vi "FGV FT-IR Kalibrieren.vi"(10 "Aktionen FT-IR Kalibrieren":T1, 11 "Sprachliste":string[][](array[string])) -> (1 "Zustand FT-IR":string, 2 "Aktionen FT-IR Kalibrieren":T1)   [LabVIEW 2020, in "Auto Kalibrieren.lvlib"]
uses:
  Auto Kalibrieren.lvlib
  Aktionen FT-IR Kalibrieren.ctl
  Seiten/FT-IR/FGV FT-IR Aktionen.ctl
  Seiten/FT-IR/FGV FT-IR Gasliste Aktionen.ctl
  Aktion FGV CalZustand.ctl
  Stoerungen/Stoerungen Messgeraet/Aktionen Kommunikation Stoerung.ctl
  Aktionen FGV Zustand Kalibrierung.ctl
  Messdaten/Aktionen FGV Messdaten.ctl
  Schedule Modul/Aktion FGV Testdaten sammeln.ctl
  Seiten/FT-IR/TOOLweb Interface Library/Trigger Aktionen.ctl
  Seiten/FT-IR/ReadLabFile/Aktionen Lab File.ctl
  Seiten/FT-IR/FT-IR.lvlib
  Allgemein/allgemeine Sub-VIs.lvlib
  Stoerungen/Stoerungen.lvlib
  Seiten/FT-IR/TOOLweb Interface Library/Typdefinitionen.lvlib
  Seiten/FT-IR/TOOLweb Interface Library/TOOLweb Interface.lvlib
  Messdaten/Messdaten.lvlib
  Seiten/FT-IR/ReadLabFile/Read Lab File.lvlib
  Sprachverwaltung/Sprachverwaltung.lvlib
  Schedule Modul/Schedule Modul.lvlib
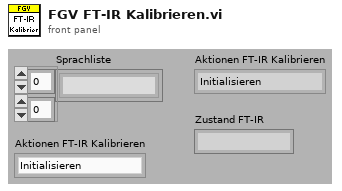
[diagram p1: front panel]
types:
  T1 = typedef "Auto Kalibrieren.lvlib/Aktionen FT-IR Kalibrieren.ctl" = enum16{"Initialisieren", "Anstehende Störung", "CO2, H2O - Vergleichen", "Hintergrund starten", "Hintergrund", "Hintergrund Abgeschlossen", "Fertig", "Beenden"}
  T2 = typedef "Auto Kalibrieren.lvlib/Aktion FGV CalZustand.ctl" = enum16{"lesen", "Cal FTIR", "Cal FID CH4", "Cal PMA", "init", "Cal FID THC", "THC CG Eingang"}
  T3 = typedef "FT-IR.lvlib/FGV FT-IR Gasliste Aktionen.ctl" = enum16{"lesen", "Gasliste FT-IR", "Gasliste ausgelesen", "laden", "speichern", "löschen"}
  T4 = typedef "FT-IR.lvlib/FGV FT-IR Aktionen.ctl" = enum16{"lesen", "NOG setzen", "NOS setzen", "Initialisieren", "speichern", "ALLES setzen", "FT-IR Spektrum loggen", "Komm Stoppen", "Spektrum LogKonfig"}
  T5 = typedef "Stoerungen.lvlib/Aktionen Kommunikation Stoerung.ctl" = enum16{"lesen", "init", "FT-IR Komm", "FT-IR Betriebsart", "FT-IR Hintergrund", "cRIO Komm", "PNS Komm", "Dichtheitstest", "Life Bit", "FTIR Komm AK", "PMA Komm", "FID Komm", "PMA Cal", "FID Ch4 Cal", "FID THC Cal", "Cal Timeout", "VFS 1 Komm", "VFS 2 Komm", "VFS 3 Komm", "VFS 4 Komm", "TRE 08 Komm", "CG-Test vorzeitig", "CG-Test Span 1", "CG-Test Span 2", "CG-Test Span 3", "CG-Test Messgas", "CG-Test löschen", "Test", "Amium AK", "AK Recept konfig", "AK Name konfig", "AK EKFG konfig"}
  T6 = typedef "Auto Kalibrieren.lvlib/Aktionen FGV Zustand Kalibrierung.ctl" = enum16{"lesen", "LÖSCHEN", "Hintergrund fertig", "Nullpunkt NDIR CO lo", "Endpunkt NDIR CO lo", "Nullpunkt NDIR CO hi", "Endpunkt NDIR CO hi", "Nullpunkt NDIR CO2 lo", "Endpunkt NDIR CO2 lo", "Nullpunkt FID CH4", "Endpunkt FID CH4", "Nullpunkt FID THC", "Endpunkt FID THC", "Nullpunkt PMA", "Endpunkt PMA", "Fehler FT-IR", "Fehler NDIR lo", "Fehler FID CH4", "Fehler FID THC", "Fehler PMA", "TIMEOUT"}
  T7 = typedef "Messdaten.lvlib/Aktionen FGV Messdaten.ctl" = enum16{"lesen", "schreiben", "löschen", "Mittelwerte", "Komponente"}
  T8 = typedef "Schedule Modul.lvlib/Aktion FGV Testdaten sammeln.ctl" = enum16{"lesen", "Dichtheitstest", "CalGasTest", "T90", "Kalibrieren", "init", "Kalender Daten"}
  T9 = typedef "FT-IR.lvlib/TOOLweb Interface.lvlib/Typdefinitionen.lvlib/Trigger Aktionen.ctl" = enum16{"startrun", "runonce", "stoprun", "pauserun", "resumerun", "takeback"}
  T10 = typedef "FT-IR.lvlib/Read Lab File.lvlib/Aktionen Lab File.ctl" = enum16{"lesen", "laden"}
  T11 = typedef "String - Ausgabefeld.ctl" = string
  T12 = typedef "Stoerungen.lvlib/Stoerungen Messgeraete.ctl" = cluster{"FT-IR Komm":bool, "FT-IR Betriebsart":bool, "FT-IR Hintergrundscan":bool, "Dichtheitstest":bool, "cRIO Komm":bool, "PNS Komm":bool, "Life Bit":bool, "FT-IR AK Komm":bool, "PMA Komm":bool, "FID Komm":bool, "PMA Cal":bool, "FID CH4 Cal":bool, "FID THC Cal":bool, "Cal Timeout":bool, "VFS 1 Komm":bool, "VFS 2 Komm":bool, "VFS 3 Komm":bool, "VFS 4 Komm":bool, "TRE 08 Komm":bool, "CG-Test":bool, "CG-Test 1":bool, "CG-Test 2":bool, "CG-Test 3":bool, "Messgas - Eingang":bool, "Amium AK Komm":bool, "AK Rezept nicht konfiguriert ":bool, "AK Name nicht konfiguriert":bool, "AK EKFG nicht konfiguriert":bool}
  T13 = typedef "Schedule Modul.lvlib/Ergebnis Kalibrieren.ctl" = cluster{"Fehler":bool, "CO2 H2O vergleich":bool}
  T14 = typedef "Auto Kalibrieren.lvlib/Zustand Messgeraete Kalibrierung.ctl" = cluster{"Hintergrund FT-IR":bool, "Nullpunkt NDIR CO lo":bool, "Endpunkt NDIR CO lo":bool, "Nullpunkt NDIR CO hi":bool, "Endpunkt NDIR CO hi":bool, "Nullpunkt NDIR CO2 lo":bool, "Endpunkt NDIR CO2 lo":bool, "Nullpunkt FID CH4":bool, "Endpunkt FID CH4":bool, "Nullpunkt FID THC":bool, "Endpunkt FID THC":bool, "Nullpunkt PMA":bool, "Endpunkt PMA":bool, "Fehler FT-IR":bool, "Fehler NDIR lo":bool, "Fehler FID CH4":bool, "Fehler FID THC":bool, "Fehler PMA":bool}
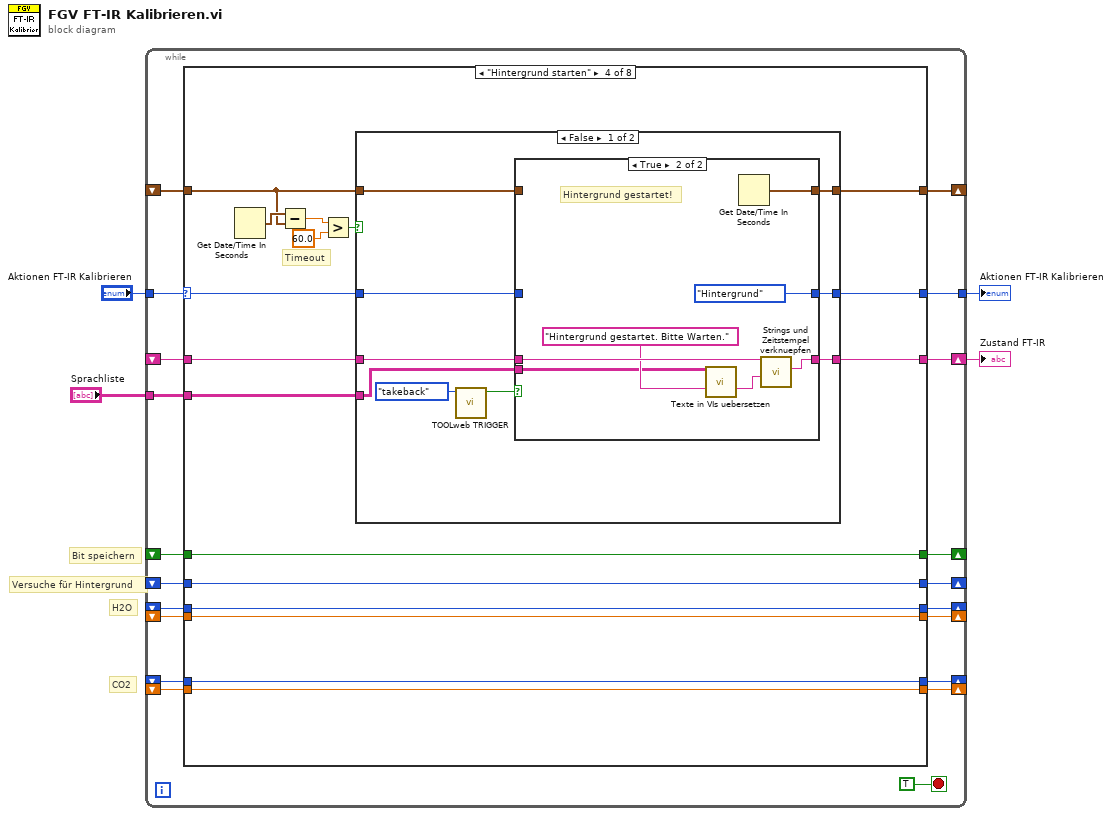
[diagram p0: block diagram]
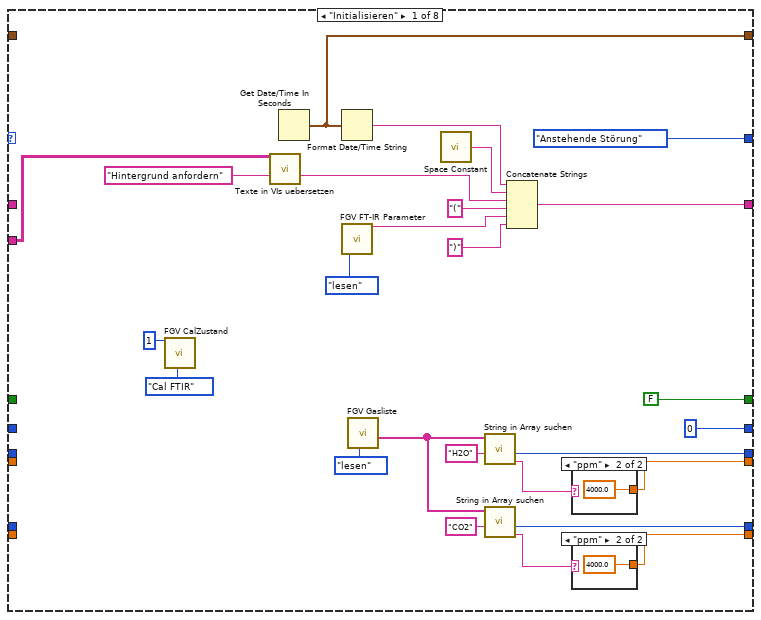
[diagram p2: hidden frame]
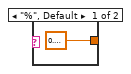
[diagram p3: hidden frame]
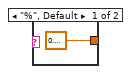
[diagram p4: hidden frame]
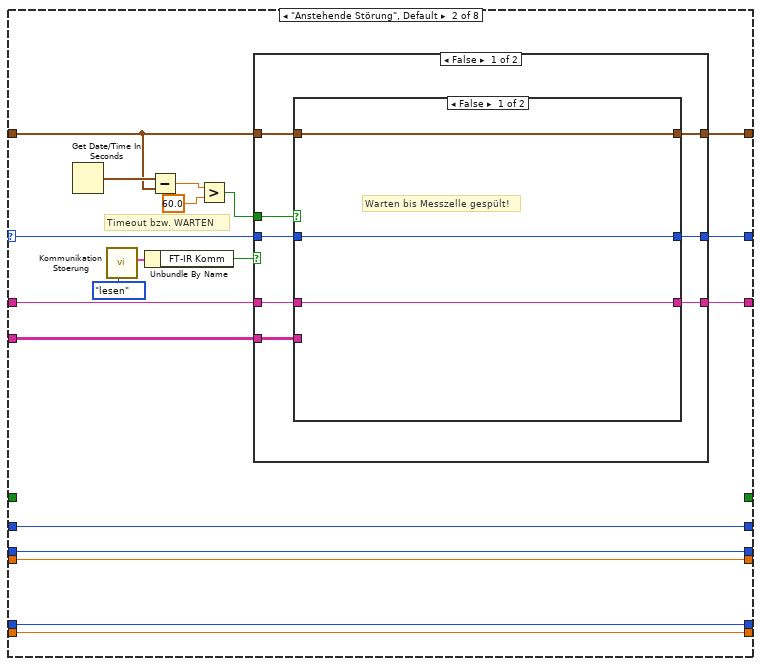
[diagram p5: hidden frame]
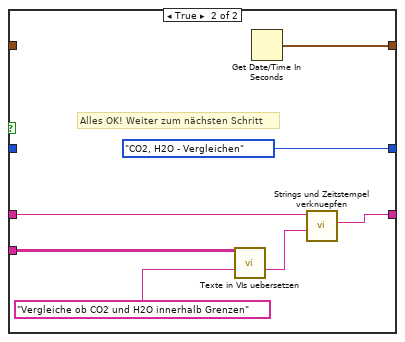
[diagram p6: hidden frame]
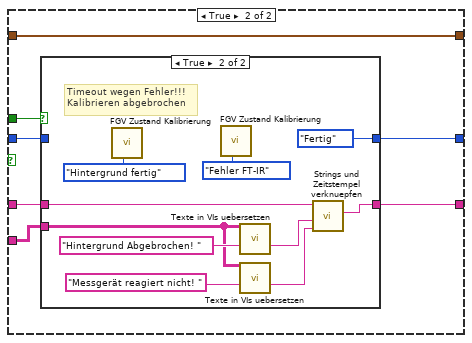
[diagram p7: hidden frame]
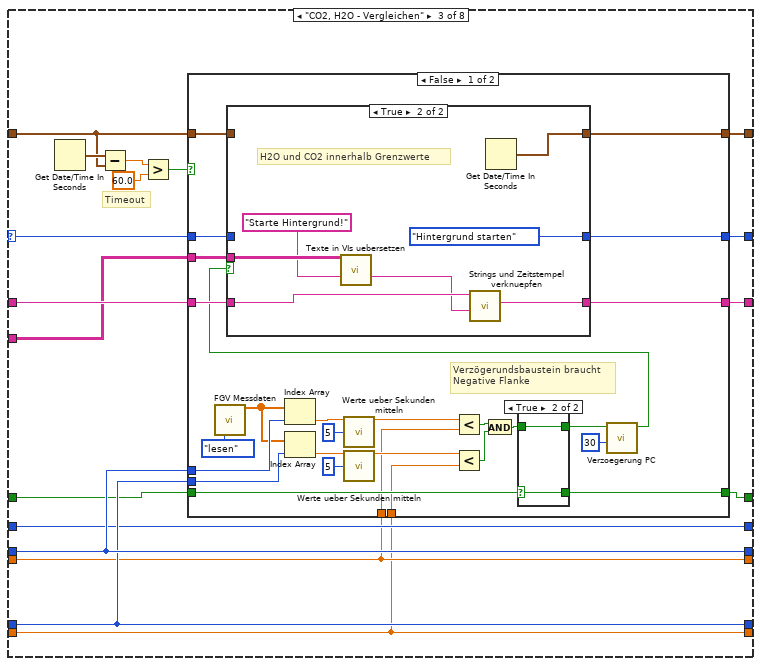
[diagram p9: hidden frame]
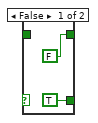
[diagram p10: hidden frame]
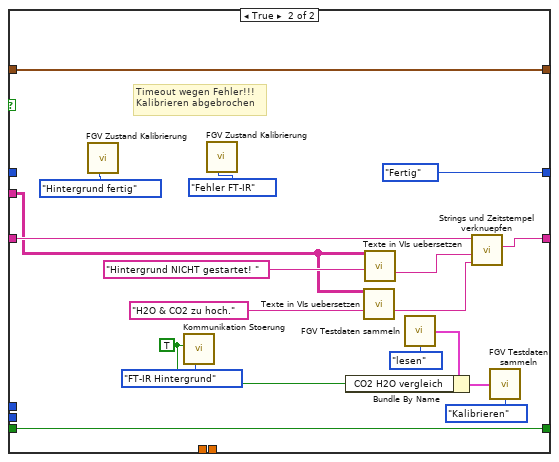
[diagram p12: hidden frame]
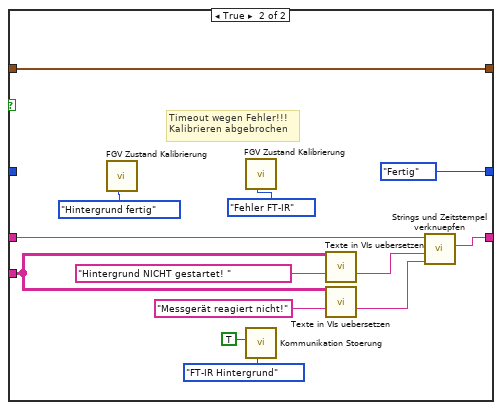
[diagram p14: hidden frame]
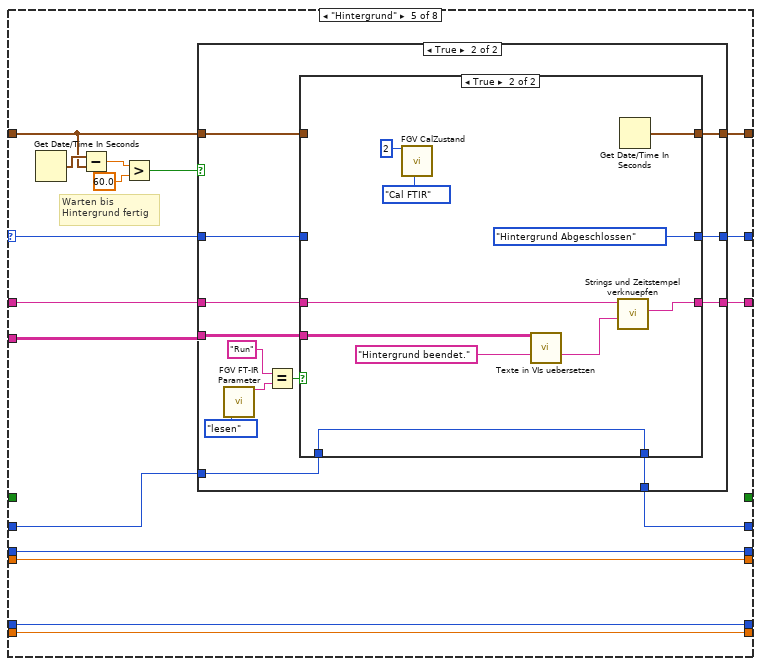
[diagram p15: hidden frame]
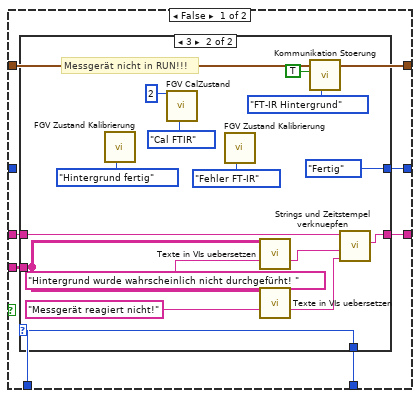
[diagram p17: hidden frame]
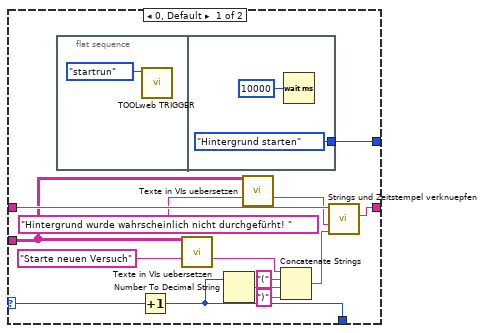
[diagram p18: hidden frame]
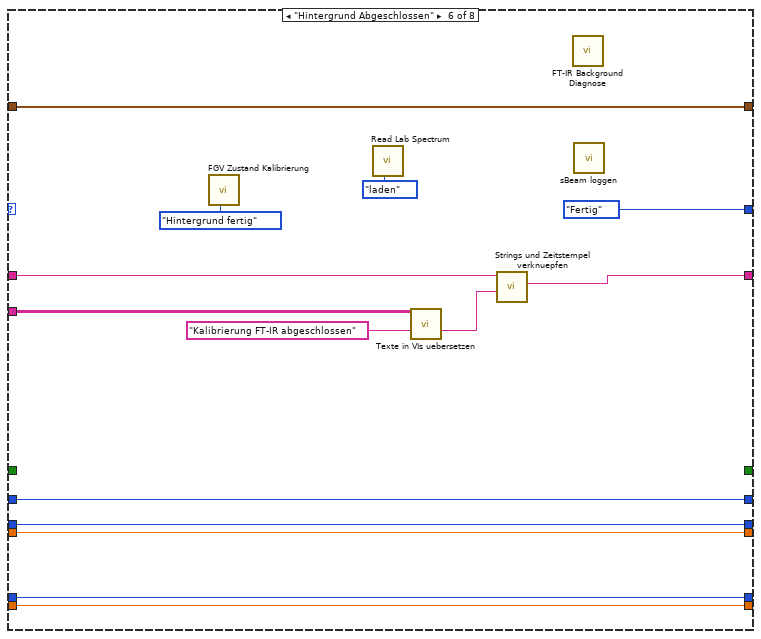
[diagram p19: hidden frame]
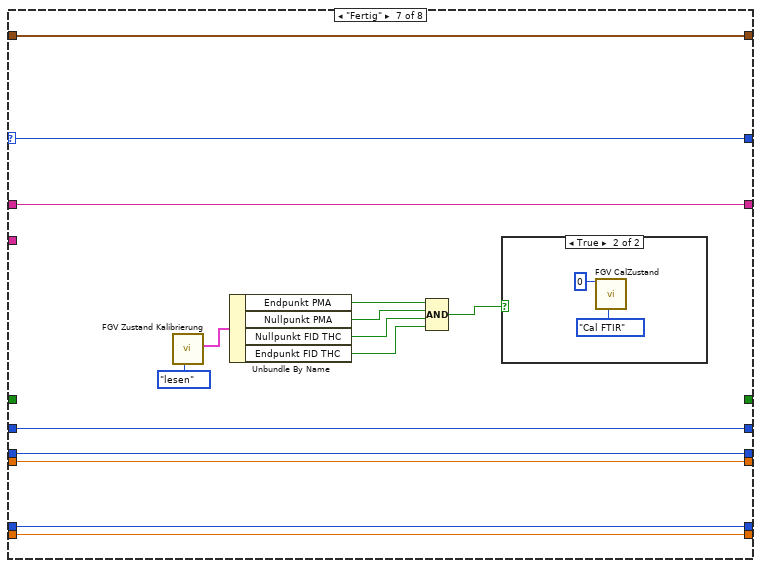
[diagram p20: hidden frame]
diagram:
  # "CO2"
  # "H2O"
  # "Versuche für Hintergrund"
  # "Bit speichern"
  n1 = while {
    shift-right: [w22] -> _
    shift-left: _ -> [w23]
    shift-right: [w18] -> w4
    shift-left: _ -> [w17]
    shift-right: [w15] -> _
    shift-left: _ -> [w20]
    shift-right: [w16] -> _
    shift-left: _ -> [w19]
    tunnel: "Aktionen FT-IR Kalibrieren" -> [w24]
    tunnel: [w21] -> w3
    shift-right: [w12] -> _
    shift-left: _ -> [w13]
    shift-right: [w11] -> _
    shift-left: _ -> [w10]
    tunnel: "Sprachliste" -> [w9]
    shift-right: [w8] -> _
    shift-left: _ -> [w7]
    shift-right: [w6] -> _
    shift-left: _ -> [w5]
    stop <- TRUE stop-if-true
    n2 = case shown="\"Hintergrund starten\"" w24 {
      selector: w24 -> [_ w66 w119 w195 w244 _ w347 _]
      tunnel: w23 -> [_ w62 w121 w196 w247 w332 w348 _]
      tunnel: [w43 w61 w120 w197 w246 w332 w348 w354] -> w22
      tunnel: [Aktionen_FT-IR_Kalibrieren."Anstehende Störung" ("Aktionen FT-IR Kalibrieren") w67 w124 w200 w248 Aktionen_FT-IR_Kalibrieren."Fertig" ("Aktionen FT-IR Kalibrieren") w347 Aktionen_FT-IR_Kalibrieren."Fertig" ("Aktionen FT-IR Kalibrieren")] -> w21
      tunnel: w17 -> [_ w64 w123 w199 w249 w331 w346 _]
      tunnel: [w42 w63 w122 w198 w245 w330 w346 "" ("Verknüpfter String")] -> w18
      tunnel: w20 -> [_ w60 w118 w194 w241 w329 w345 w358]
      tunnel: w19 -> [_ w59 w117 w193 w240 w328 w344 w357]
      tunnel: [w29 w59 w117 w193 w240 w328 w344 w357] -> w16
      tunnel: [w30 w60 w118 w194 w241 w329 w345 w358] -> w15
      tunnel: w13 -> [_ _ w116 w192 _ _ _ _]
      tunnel: [FALSE _ w115 w192 _ _ _ _] -> w12
      tunnel: [u16 0 w58 w114 w191 w242 w326 w340 w353] -> w11
      tunnel: w10 -> [_ w58 w114 w191 w243 w326 w340 w353]
      tunnel: w9 -> [w33 w57 w113 w190 w239 w322 _ _]
      tunnel: [w27 w56 w112 w189 w238 w321 w335 w352] -> w8
      tunnel: w7 -> [_ w56 w112 w189 w238 w321 w335 w352]
      tunnel: [w25 w55 w111 w188 w237 w320 w334 w351] -> w6
      tunnel: w5 -> [_ w55 w111 w188 w237 w320 w334 w351]
      frame "Initialisieren" {
        n3 = call "FGV CalZustand.vi"("CAL Zustand"=u16 1 ("CAL Zustand FTIR"), "Aktion"=Aktion_FGV_CalZustand."Cal FTIR") -> ()  [unwired: 13 in, 5 out]
        n4 = call "Texte in VIs uebersetzen.vi"("Sprachliste"=w33, "String zum Übersetzen"="Hintergrund anfordern" ("String")) -> ("String zum Übersetzen"=w31:string)  [unwired: 9 in, 4 out]
        n5 = Get Date/Time In Seconds() -> (seconds since 1Jan1904=w43:timestamp)
        n6 = Format Date/Time String(seconds (now)=w43) -> (date/time string=w44:string)  [unwired: 2 in]
        n7 = call "FGV FT-IR Parameter.vi"("Aktion"=FGV_FT-IR_Aktionen."lesen") -> ("Instrument State"=w47:string)  [unwired: 11 in, 7 out]
        n8 = call "FGV Gasliste.vi"("Aktionen"=FGV_FT-IR_Gasliste_Aktionen."lesen") -> ("Aktuelle Gasliste gesamt"=w37:T11[])  [unwired: 8 in, 2 out]
        n9 = call <vilib>:"Space Constant.vi"() -> ("String"=w49:string)
        n10 = call "String in Array suchen.vi"("Nach String/Zeichen suchen (-)"="H2O", "String-Array"=w37) -> ("Einheit"=w28:string, "Index"=w30:i32)  [unwired: 7 in, 1 out]
        n11 = call "String in Array suchen.vi"("Nach String/Zeichen suchen (-)"="CO2", "String-Array"=w37) -> ("Einheit"=w26:string, "Index"=w29:i32)  [unwired: 7 in, 1 out]
        n12 = Concatenate Strings(w44, w49, w31, "(" ("String"), w47, ")" ("String")) -> (w42:string)
        n13 = case shown="\"ppm\"" w28 {
          tunnel: [sgl 0.4 ("y") sgl 4000.0 ("y")] -> w27
          frame "%", Default {
          }
          frame "ppm" {
          }
        }
        n14 = case shown="\"ppm\"" w26 {
          tunnel: [sgl 0.4 ("y") sgl 4000.0 ("y")] -> w25
          frame "%", Default {
          }
          frame "ppm" {
          }
        }
      }
      frame "Anstehende Störung", Default {
        # "Timeout bzw. WARTEN"
        n15 = Get Date/Time In Seconds() -> (seconds since 1Jan1904=w70:timestamp)
        n16 = call "Kommunikation Stoerung.vi"("Aktionen"=Aktionen_Kommunikation_Stoerung."lesen") -> ("Störung Messgerät"=w72:T12)  [unwired: 2 in, 8 out]
        n17 = Unbundle By Name(w72) -> ("FT-IR Komm"=w71:bool)
        n18 = Subtract(x=w70, y=w62) -> (x-y=w69:dbl)
        n19 = Greater?(x=w69, y=60.0) -> (0:w65:bool)
        n20 = case shown="False" w71 {
          tunnel: [w81 w96] -> w67
          tunnel: w66 -> [w75 w97]
          tunnel: w65 -> [w77 w98]
          tunnel: w64 -> [w79 w95]
          tunnel: [w78 w94] -> w63
          tunnel: w62 -> [w76 w93]
          tunnel: [w80 w93] -> w61
          tunnel: w57 -> [w74 w92]
          frame False {
            n21 = case shown="False" w77 {
              tunnel: [w83 Aktionen_FT-IR_Kalibrieren."CO2, H2O - Vergleichen" ("Aktionen FT-IR Kalibrieren")] -> w81
              tunnel: [w84 w90] -> w80
              tunnel: w79 -> [w82 w89]
              tunnel: [w82 w88] -> w78
              tunnel: w76 -> [w84 _]
              tunnel: w75 -> [w83 _]
              tunnel: w74 -> [_ w87]
              frame False {
                # "Warten bis Messzelle gespült!"
              }
              frame True {
                # "Alles OK! Weiter zum nächsten Schritt"
                n22 = call "Texte in VIs uebersetzen.vi"("Sprachliste"=w87, "String zum Übersetzen"="Vergleiche ob CO2 und H2O innerhalb Grenzen" ("String")) -> ("String zum Übersetzen"=w86:string)  [unwired: 9 in, 4 out]
                n23 = Get Date/Time In Seconds() -> (seconds since 1Jan1904=w90:timestamp)
                n24 = call "Strings und Zeitstempel verknuepfen.vi"("String 1 hinzufügen"=w86, "Eingagns String"=w89) -> ("Verknüpfter String"=w88:string)  [unwired: 9 in]
              }
            }
          }
          frame True {
            n25 = case shown="True" w98 {
              tunnel: w97 -> [w100 _]
              tunnel: [w100 Aktionen_FT-IR_Kalibrieren."Fertig" ("Aktionen FT-IR Kalibrieren")] -> w96
              tunnel: w95 -> [w99 w109]
              tunnel: [w99 w108] -> w94
              tunnel: w92 -> [_ w103]
              frame False {
                # "Fehler steht an!!!!"
              }
              frame True {
                # "Timeout wegen Fehler!!! \nKalibrieren abgebrochen"
                n26 = call "FGV Zustand Kalibrierung.vi"("Aktionen"=Aktionen_FGV_Zustand_Kalibrierung."Hintergrund fertig" ("Enum")) -> ()  [unwired: 9 in, 2 out]
                n27 = call "FGV Zustand Kalibrierung.vi"("Aktionen"=Aktionen_FGV_Zustand_Kalibrierung."Fehler FT-IR" ("Enum")) -> ()  [unwired: 9 in, 2 out]
                n28 = call "Texte in VIs uebersetzen.vi"("Sprachliste"=w103, "String zum Übersetzen"="Hintergrund Abgebrochen! " ("String")) -> ("String zum Übersetzen"=w104:string)  [unwired: 9 in, 4 out]
                n29 = call "Texte in VIs uebersetzen.vi"("Sprachliste"=w103, "String zum Übersetzen"="Messgerät reagiert nicht! " ("String")) -> ("String zum Übersetzen"=w102:string)  [unwired: 9 in, 4 out]
                n30 = call "Strings und Zeitstempel verknuepfen.vi"("String 2 hinzufügen"=w102, "String 1 hinzufügen"=w104, "Eingagns String"=w109) -> ("Verknüpfter String"=w108:string)  [unwired: 8 in]
              }
            }
          }
        }
      }
      frame "CO2, H2O - Vergleichen" {
        # "Timeout"
        n31 = Get Date/Time In Seconds() -> (seconds since 1Jan1904=w128:timestamp)
        n32 = Subtract(x=w128, y=w121) -> (x-y=w127:dbl)
        n33 = Greater?(x=w127, y=60.0) -> (0:w125:bool)
        n34 = case shown="False" w125 {
          tunnel: [w149 Aktionen_FT-IR_Kalibrieren."Fertig" ("Aktionen FT-IR Kalibrieren")] -> w124
          tunnel: w123 -> [w151 w185]
          tunnel: [w150 w184] -> w122
          tunnel: w117 -> [w153 _]
          tunnel: w118 -> [w152 _]
          tunnel: w121 -> [w147 w186]
          tunnel: [w146 w186] -> w120
          tunnel: w119 -> [w148 _]
          tunnel: w116 -> [w142 w182]
          tunnel: [w139 w182] -> w115
          tunnel: w113 -> [w138 w175]
          tunnel: w112 -> [w130 _]
          tunnel: w111 -> [w129 _]
          frame False {
            # "Verzögerundsbaustein braucht\nNegative Flanke"
            n35 = call "FGV Messdaten.vi"("Aktionen"=Aktionen_FGV_Messdaten."lesen") -> ("Aktuelle Messwerte"=w137:sgl[])  [unwired: 6 in, 8 out]
            n36 = Index Array(array=w137, index=w152) -> (element=w155:sgl)
            n37 = Index Array(array=w137, index=w153) -> (element=w154:sgl)
            n38 = call "Werte ueber Sekunden mitteln.vi"("Neuer Wert"=w155, "Sek"=u32 5) -> ("gemittelter Wert"=w134:sgl)  [unwired: 12 in, 1 out]
            n39 = call "Werte ueber Sekunden mitteln.vi"("Neuer Wert"=w154, "Sek"=u32 5) -> ("gemittelter Wert"=w133:sgl)  [unwired: 12 in, 1 out]
            n40 = Less?(x=w134, y=w130) -> (x < y?=w132:bool)
            n41 = Less?(x=w133, y=w129) -> (x < y?=w131:bool)
            n42 = And(x=w132, y=w131) -> (x .and. y?=w144:bool)
            n43 = case shown="True" w142 {
              selector: w142 -> [_ w159]
              tunnel: w144 -> [_ w158]
              tunnel: [FALSE w158] -> w143
              tunnel: [TRUE w159] -> w139
              frame False {
              }
              frame True {
              }
            }
            n44 = call "Verzoegerung PC.vi"("sec"=u16 30, "Startsignal"=w143) -> ("Zeit abgelaufen?"=w140:bool)  [unwired: 8 in, 1 out]
            n45 = case shown="True" w140 {
              tunnel: w151 -> [w162 w167]
              tunnel: [w162 w166] -> w150
              tunnel: [w161 Aktionen_FT-IR_Kalibrieren."Hintergrund starten" ("Aktionen FT-IR Kalibrieren")] -> w149
              tunnel: w148 -> [w161 _]
              tunnel: w147 -> [w160 _]
              tunnel: [w160 w168] -> w146
              tunnel: w138 -> [_ w165]
              frame False {
                # "H2O und CO2 NICHT innerhalb Grenzwerte"
              }
              frame True {
                # "H2O und CO2 innerhalb Grenzwerte"
                n46 = call "Texte in VIs uebersetzen.vi"("Sprachliste"=w165, "String zum Übersetzen"="Starte Hintergrund!" ("String")) -> ("String zum Übersetzen"=w164:string)  [unwired: 9 in, 4 out]
                n47 = call "Strings und Zeitstempel verknuepfen.vi"("String 1 hinzufügen"=w164, "Eingagns String"=w167) -> ("Verknüpfter String"=w166:string)  [unwired: 9 in]
                n48 = Get Date/Time In Seconds() -> (seconds since 1Jan1904=w168:timestamp)
              }
            }
          }
          frame True {
            w171 = TRUE ("ERROR")
            # "Timeout wegen Fehler!!! \nKalibrieren abgebrochen"
            n49 = call "FGV Zustand Kalibrierung.vi"("Aktionen"=Aktionen_FGV_Zustand_Kalibrierung."Hintergrund fertig" ("Enum")) -> ()  [unwired: 9 in, 2 out]
            n50 = call "Kommunikation Stoerung.vi"("Aktionen"=Aktionen_Kommunikation_Stoerung."FT-IR Hintergrund", "ERROR"=w171) -> ()  [unwired: 9 in, 1 out]
            n51 = call "FGV Zustand Kalibrierung.vi"("Aktionen"=Aktionen_FGV_Zustand_Kalibrierung."Fehler FT-IR" ("Enum")) -> ()  [unwired: 9 in, 2 out]
            n52 = call "Texte in VIs uebersetzen.vi"("Sprachliste"=w175, "String zum Übersetzen"="H2O & CO2 zu hoch." ("String")) -> ("String zum Übersetzen"=w176:string)  [unwired: 9 in, 4 out]
            n53 = call "Texte in VIs uebersetzen.vi"("Sprachliste"=w175, "String zum Übersetzen"="Hintergrund NICHT gestartet! " ("String")) -> ("String zum Übersetzen"=w178:string)  [unwired: 9 in, 4 out]
            n54 = call "FGV Testdaten sammeln.vi"("Aktion"=Aktion_FGV_Testdaten_sammeln."lesen") -> ("Ergebnisse Kalibrieren"=w173:T13)  [unwired: 9 in, 5 out]
            n55 = Bundle By Name(cluster=w173, "CO2 H2O vergleich"=w171) -> (w172:T13)
            n56 = call "Strings und Zeitstempel verknuepfen.vi"("String 2 hinzufügen"=w176, "String 1 hinzufügen"=w178, "Eingagns String"=w185) -> ("Verknüpfter String"=w184:string)  [unwired: 8 in]
            n57 = call "FGV Testdaten sammeln.vi"("Ergebnisse Kalibrieren"=w172, "Aktion"=Aktion_FGV_Testdaten_sammeln."Kalibrieren") -> ()  [unwired: 8 in, 6 out]
          }
        }
      }
      frame "Hintergrund starten" {
        # "Timeout"
        n58 = Get Date/Time In Seconds() -> (seconds since 1Jan1904=w204:timestamp)
        n59 = Subtract(x=w204, y=w196) -> (x-y=w203:dbl)
        n60 = Greater?(x=w203, y=60.0) -> (0:w201:bool)
        n61 = case shown="False" w201 {
          tunnel: [w212 Aktionen_FT-IR_Kalibrieren."Fertig" ("Aktionen FT-IR Kalibrieren")] -> w200
          tunnel: w199 -> [w211 w234]
          tunnel: [w208 w233] -> w198
          tunnel: [w209 w235] -> w197
          tunnel: w196 -> [w210 w235]
          tunnel: w195 -> [w213 _]
          tunnel: w190 -> [w205 w224]
          frame False {
            n62 = call "TOOLweb TRIGGER.vi"("action"=Trigger_Aktionen."takeback") -> ("Trigger ausgeführt"=w206:bool)  [unwired: 5 in, 1 out]
            n63 = case shown="True" w206 {
              tunnel: w213 -> [w216 _]
              tunnel: [w216 Aktionen_FT-IR_Kalibrieren."Hintergrund" ("Aktionen FT-IR Kalibrieren")] -> w212
              tunnel: w211 -> [w215 w223]
              tunnel: w210 -> [w214 _]
              tunnel: [w214 w220] -> w209
              tunnel: [w215 w222] -> w208
              tunnel: w205 -> [_ w217]
              frame False {
                # "Keine Kommunikation zu Messgerät"
              }
              frame True {
                # "Hintergrund gestartet!"
                n64 = call "Texte in VIs uebersetzen.vi"("Sprachliste"=w217, "String zum Übersetzen"="Hintergrund gestartet. Bitte Warten." ("String")) -> ("String zum Übersetzen"=w218:string)  [unwired: 9 in, 4 out]
                n65 = Get Date/Time In Seconds() -> (seconds since 1Jan1904=w220:timestamp)
                n66 = call "Strings und Zeitstempel verknuepfen.vi"("String 1 hinzufügen"=w218, "Eingagns String"=w223) -> ("Verknüpfter String"=w222:string)  [unwired: 9 in]
              }
            }
          }
          frame True {
            # "Timeout wegen Fehler!!! \nKalibrieren abgebrochen"
            n67 = call "FGV Zustand Kalibrierung.vi"("Aktionen"=Aktionen_FGV_Zustand_Kalibrierung."Hintergrund fertig" ("Enum")) -> ()  [unwired: 9 in, 2 out]
            n68 = call "FGV Zustand Kalibrierung.vi"("Aktionen"=Aktionen_FGV_Zustand_Kalibrierung."Fehler FT-IR" ("Enum")) -> ()  [unwired: 9 in, 2 out]
            n69 = call "Kommunikation Stoerung.vi"("Aktionen"=Aktionen_Kommunikation_Stoerung."FT-IR Hintergrund", "ERROR"=TRUE) -> ()  [unwired: 9 in, 1 out]
            n70 = call "Texte in VIs uebersetzen.vi"("Sprachliste"=w224, "String zum Übersetzen"="Hintergrund NICHT gestartet! " ("String")) -> ("String zum Übersetzen"=w227:string)  [unwired: 9 in, 4 out]
            n71 = call "Texte in VIs uebersetzen.vi"("Sprachliste"=w224, "String zum Übersetzen"="Messgerät reagiert nicht!" ("String")) -> ("String zum Übersetzen"=w225:string)  [unwired: 9 in, 4 out]
            n72 = call "Strings und Zeitstempel verknuepfen.vi"("String 2 hinzufügen"=w225, "String 1 hinzufügen"=w227, "Eingagns String"=w234) -> ("Verknüpfter String"=w233:string)  [unwired: 8 in]
          }
        }
      }
      frame "Hintergrund" {
        # "Warten bis \nHintergrund fertig"
        n73 = Get Date/Time In Seconds() -> (seconds since 1Jan1904=w253:timestamp)
        n74 = Subtract(x=w253, y=w247) -> (x-y=w252:dbl)
        n75 = Greater?(x=w252, y=60.0) -> (0:w250:bool)
        n76 = case shown="True" w250 {
          tunnel: w249 -> [w255 w264]
          tunnel: [w256 w265] -> w248
          tunnel: w247 -> [w257 w267]
          tunnel: [w257 w266] -> w246
          tunnel: [w255 w263] -> w245
          tunnel: w244 -> [w256 w262]
          tunnel: w243 -> [w254 w260]
          tunnel: [w254 w259] -> w242
          tunnel: w239 -> [_ w258]
          frame False {
          }
          frame True {
            n77 = call "FGV FT-IR Parameter.vi"("Aktion"=FGV_FT-IR_Aktionen."lesen") -> ("Instrument State"=w269:string)  [unwired: 11 in, 7 out]
            n78 = Equal?(x="Run", y=w269) -> (x = y?=w261:bool)
            n79 = case shown="True" w261 {
              tunnel: w267 -> [w277 _]
              tunnel: [w277 w319] -> w266
              tunnel: [w276 Aktionen_FT-IR_Kalibrieren."Hintergrund Abgeschlossen" ("Aktionen FT-IR Kalibrieren")] -> w265
              tunnel: w264 -> [w274 w317]
              tunnel: [w275 w316] -> w263
              tunnel: w262 -> [_ _]
              tunnel: w260 -> [w273 w315]
              tunnel: [w272 w315] -> w259
              tunnel: w258 -> [w271 w310]
              frame False {
                n80 = case shown="3" w273 {
                  selector: w273 -> [w288 w303]
                  tunnel: [w289 Aktionen_FT-IR_Kalibrieren."Fertig" ("Aktionen FT-IR Kalibrieren")] -> w276
                  tunnel: [w291 w308] -> w275
                  tunnel: w274 -> [w290 w307]
                  tunnel: [w283 w303] -> w272
                  tunnel: w271 -> [w278 w295]
                  frame 0, Default {
                    n81 = flat-sequence {
                      tunnel: [Aktionen_FT-IR_Kalibrieren."Hintergrund starten" ("Aktionen FT-IR Kalibrieren")] -> w289
                      frame #0 {
                        n82 = call "TOOLweb TRIGGER.vi"("action"=Trigger_Aktionen."startrun") -> ()  [unwired: 5 in, 2 out]
                      }
                      frame #1 {
                        n83 = Wait (ms)(milliseconds to wait=u32 10000 ("Zu wartende ms")) -> ()  [unwired: 1 out]
                      }
                    }
                    n84 = Increment(x=w288) -> (x+1=w283:u16)
                    n85 = call "Texte in VIs uebersetzen.vi"("Sprachliste"=w278, "String zum Übersetzen"="Starte neuen Versuch" ("String")) -> ("String zum Übersetzen"=w279:string)  [unwired: 9 in, 4 out]
                    n86 = Number To Decimal String(number=w283) -> (decimal integer string=w286:string)  [unwired: 1 in]
                    n87 = call "Texte in VIs uebersetzen.vi"("Sprachliste"=w278, "String zum Übersetzen"="Hintergrund wurde wahrscheinlich nicht durchgefürht! " ("String")) -> ("String zum Übersetzen"=w281:string)  [unwired: 9 in, 4 out]
                    n88 = Concatenate Strings(w279, "(" ("String"), w286, ")" ("String")) -> (w284:string)
                    n89 = call "Strings und Zeitstempel verknuepfen.vi"("String 2 hinzufügen"=w284, "String 1 hinzufügen"=w281, "Eingagns String"=w290) -> ("Verknüpfter String"=w291:string)  [unwired: 8 in]
                  }
                  frame 3 {
                    # "Messgerät nicht in RUN!!!"
                    n90 = call "FGV Zustand Kalibrierung.vi"("Aktionen"=Aktionen_FGV_Zustand_Kalibrierung."Hintergrund fertig" ("Enum")) -> ()  [unwired: 9 in, 2 out]
                    n91 = call "FGV CalZustand.vi"("CAL Zustand"=u16 2 ("CAL Zustand FTIR"), "Aktion"=Aktion_FGV_CalZustand."Cal FTIR") -> ()  [unwired: 13 in, 5 out]
                    n92 = call "FGV Zustand Kalibrierung.vi"("Aktionen"=Aktionen_FGV_Zustand_Kalibrierung."Fehler FT-IR" ("Enum")) -> ()  [unwired: 9 in, 2 out]
                    n93 = call "Texte in VIs uebersetzen.vi"("Sprachliste"=w295, "String zum Übersetzen"="Hintergrund wurde wahrscheinlich nicht durchgefürht! " ("String")) -> ("String zum Übersetzen"=w298:string)  [unwired: 9 in, 4 out]
                    n94 = call "Texte in VIs uebersetzen.vi"("Sprachliste"=w295, "String zum Übersetzen"="Messgerät reagiert nicht!" ("String")) -> ("String zum Übersetzen"=w297:string)  [unwired: 9 in, 4 out]
                    n95 = call "Kommunikation Stoerung.vi"("Aktionen"=Aktionen_Kommunikation_Stoerung."FT-IR Hintergrund", "ERROR"=TRUE) -> ()  [unwired: 9 in, 1 out]
                    n96 = call "Strings und Zeitstempel verknuepfen.vi"("String 2 hinzufügen"=w297, "String 1 hinzufügen"=w298, "Eingagns String"=w307) -> ("Verknüpfter String"=w308:string)  [unwired: 8 in]
                  }
                }
              }
              frame True {
                n97 = call "FGV CalZustand.vi"("CAL Zustand"=u16 2 ("CAL Zustand FTIR"), "Aktion"=Aktion_FGV_CalZustand."Cal FTIR") -> ()  [unwired: 13 in, 5 out]
                n98 = call "Texte in VIs uebersetzen.vi"("Sprachliste"=w310, "String zum Übersetzen"="Hintergrund beendet." ("String")) -> ("String zum Übersetzen"=w311:string)  [unwired: 9 in, 4 out]
                n99 = call "Strings und Zeitstempel verknuepfen.vi"("String 1 hinzufügen"=w311, "Eingagns String"=w317) -> ("Verknüpfter String"=w316:string)  [unwired: 9 in]
                n100 = Get Date/Time In Seconds() -> (seconds since 1Jan1904=w319:timestamp)
              }
            }
          }
        }
      }
      frame "Hintergrund Abgeschlossen" {
        n101 = call "FGV Zustand Kalibrierung.vi"("Aktionen"=Aktionen_FGV_Zustand_Kalibrierung."Hintergrund fertig" ("Enum")) -> ()  [unwired: 9 in, 2 out]
        n102 = call "Read Lab Spectrum.VI"("Aktionen"=Aktionen_Lab_File."laden") -> ()  [unwired: 7 in, 4 out]
        n103 = call "Texte in VIs uebersetzen.vi"("Sprachliste"=w322, "String zum Übersetzen"="Kalibrierung FT-IR abgeschlossen" ("String")) -> ("String zum Übersetzen"=w323:string)  [unwired: 9 in, 4 out]
        n104 = call "Strings und Zeitstempel verknuepfen.vi"("String 1 hinzufügen"=w323, "Eingagns String"=w331) -> ("Verknüpfter String"=w330:string)  [unwired: 9 in]
        n105 = call "FT-IR Background Diagnose.vi"() -> ()  [unwired: 12 in]
        n106 = call "sBeam loggen.vi"() -> ()  [unwired: 11 in, 1 out]
      }
      frame "Fertig" {
        n107 = call "FGV Zustand Kalibrierung.vi"("Aktionen"=Aktionen_FGV_Zustand_Kalibrierung."lesen" ("Enum")) -> ("Zustand Kalibrierung"=w342:T14)  [unwired: 9 in, 1 out]
        n108 = Unbundle By Name(w342) -> ("Endpunkt PMA"=w339:bool, "Nullpunkt PMA"=w338:bool, "Nullpunkt FID THC"=w337:bool, "Endpunkt FID THC"=w336:bool)
        n109 = Compound Arithmetic op=AND(w339, w338, w337, w336) -> (w341:bool)
        n110 = case shown="True" w341 {
          frame False {
          }
          frame True {
            n111 = call "FGV CalZustand.vi"("CAL Zustand"=u16 0 ("CAL Zustand FTIR"), "Aktion"=Aktion_FGV_CalZustand."Cal FTIR") -> ()  [unwired: 13 in, 5 out]
          }
        }
      }
      frame "Beenden" {
        n112 = Get Date/Time In Seconds() -> (seconds since 1Jan1904=w354:timestamp)
      }
    }
  }
  "Zustand FT-IR" <- w4
  "Aktionen FT-IR Kalibrieren" <- w3
